vi "Read Coordinate Max.vi"(8 "error in (no error)":errorcluster, 11 "TSP Class in":refnum<class "TSP Class.lvclass">) -> (0 "error out":errorcluster, 2 "Coordinate Max":dbl=15.0, 3 "TSP Class out":refnum<class "TSP Class.lvclass">)   [LabVIEW 2015, in "TSP Library.lvlib" / "TSP Class.lvclass"]
uses:
  TSP Class.lvclass
  TSP Class.lvclass/TSP Class.ctl
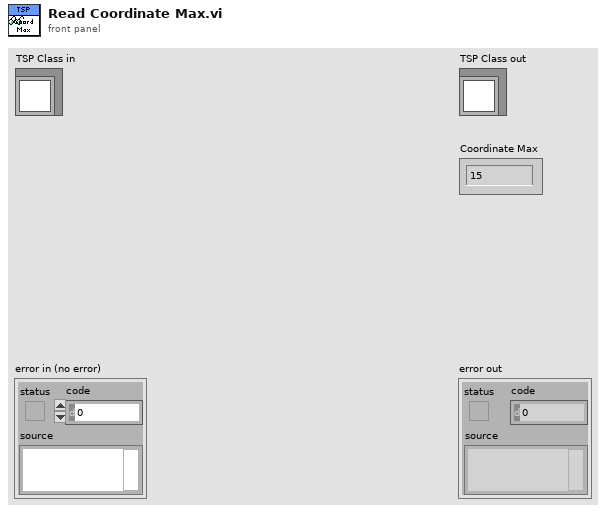
[diagram p1: front panel]
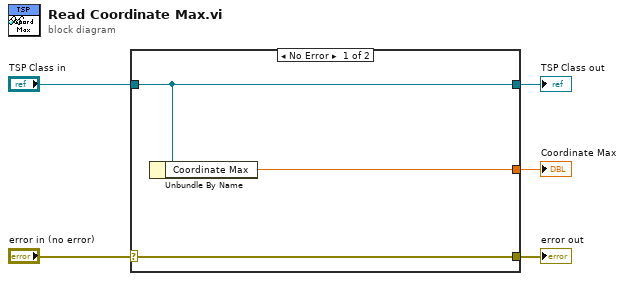
[diagram p0: block diagram]
diagram:
  n1 = case shown="No Error" "error in (no error)" {
    selector: "error in (no error)" -> [w8 w9]
    tunnel: [w8 w9] -> w4
    tunnel: [w7 w10] -> w2
    tunnel: "TSP Class in" -> [w7 w10]
    tunnel: [w6 _] -> w1
    frame No Error {
      n2 = Unbundle By Name(w7) -> ("Coordinate Max"=w6:dbl)
    }
    frame Error {
    }
  }
  "error out" <- w4
  "TSP Class out" <- w2
  "Coordinate Max" <- w1
